vi "compare_and_count.vi"(9 "count_input":i32, 10 "数值 2":i32, 11 "数值1":i32) -> (2 "count_output":i32)   [LabVIEW 2014]
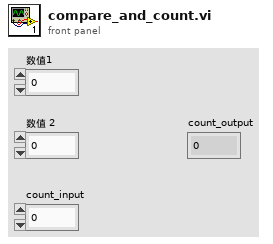
[diagram p1: front panel]
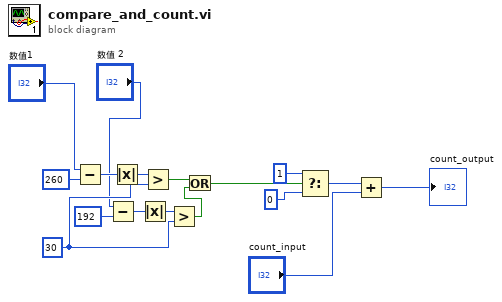
[diagram p0: block diagram]
diagram:
  w11 = 30
  n1 = Subtract(x="数值1", y=260) -> (x-y=w15:i32)
  n2 = Subtract(x="数值 2", y=192) -> (x-y=w14:i32)
  n3 = Absolute Value(x=w15) -> (abs(x)=w13:i32)
  n4 = Absolute Value(x=w14) -> (abs(x)=w12:i32)
  n5 = Greater?(x=w13, y=w11) -> (0:w10:bool)
  n6 = Greater?(x=w12, y=w11) -> (0:w9:bool)
  n7 = Or(x=w10, y=w9) -> (x .or. y?=w4:bool)
  n8 = Select(t=1, s=w4, f=0) -> (s? t:f=w3:i32)
  n9 = Add(x=w3, y="count_input") -> (x+y=→"count_output":i32)
